vi "GyroDrive.vi"(0 "X axis value":dbl, 1 "Y axis value":dbl, 2 "RobotDriveDevRef_In":T1={"DevStatus"={"status"=FALSE, "code"=0, "source"=""}, "Motors[]"=[], "Square Inputs"=FALSE, "Max Output"=1.0}, 3 "Use gyro":bool, 4 "error in (no error)":errorcluster) -> (5 "Motor Values":dbl[](array[numeric]), 6 "RobotDriveDevRef_Out":T1={"DevStatus"={"status"=FALSE, "code"=0, "source"=""}, "Motors[]"=[], "Square Inputs"=FALSE, "Max Output"=1.0}, 7 "error out":errorcluster)   [LabVIEW 2015]
uses:
  <vilib>/Rock Robotics/WPI/RobotDrive/WPI_RobotDriveDevRef.ctl
  <vilib>/Rock Robotics/WPI/MotorControl/WPI_MotorControlDeviceRef.ctl
  <vilib>/Rock Robotics/WPI/MotorControl/WPI_MotorControlType.ctl
  <vilib>/Rock Robotics/SystemInterfaces/DIO/FPGA_DIOPWMChannel.ctl
  <vilib>/Rock Robotics/WPI/PWM/WPI_PWMDeadband.ctl
  <vilib>/Rock Robotics/WPI/CAN/Jaguar/SubVIs/WPI_CANJaguar_ControlMode.ctl
  <vilib>/Rock Robotics/WPI/CAN/TalonSRX/WPI_CANTalonSRX_APIControlMode.ctl
  Robot Global Data.vi
  <vilib>/Rock Robotics/WPI/RobotDrive/WPI_RobotDriveArcadeDrive_Standard(NoSaturation).vi
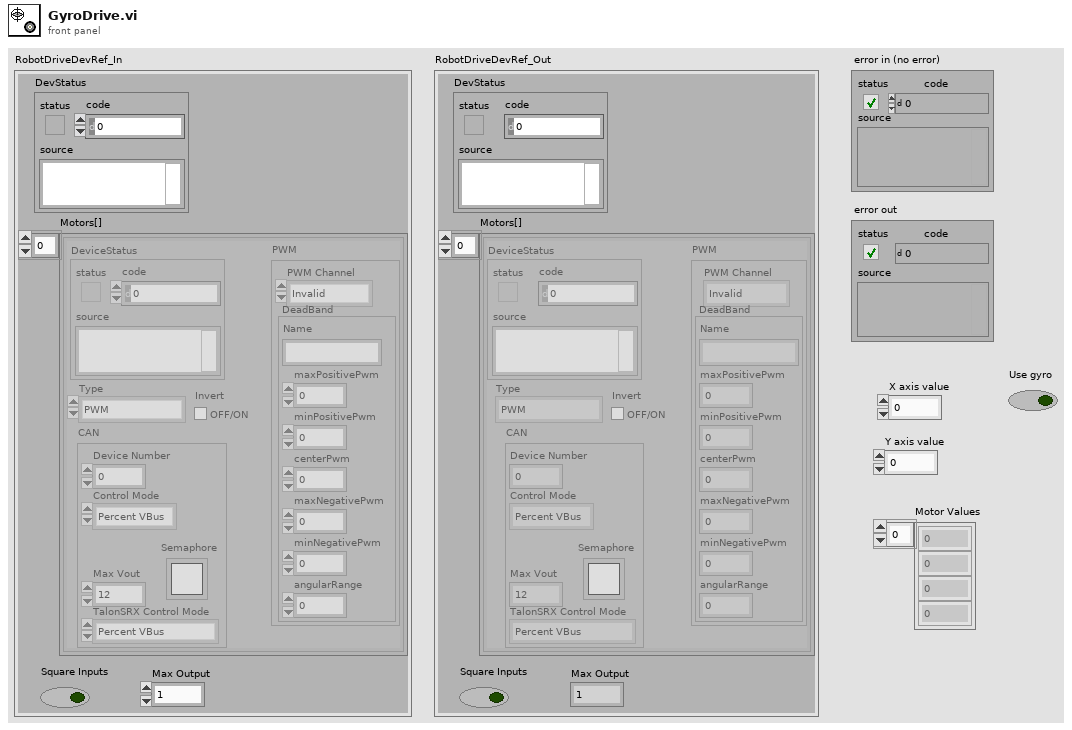
[diagram p1: front panel]
types:
  T1 = typedef "WPI_RobotDriveDevRef.ctl" = cluster{"DevStatus":errorcluster, "Motors[]":T2[], "Square Inputs":bool, "Max Output":dbl}
  T2 = typedef "WPI_MotorControlDeviceRef.ctl" = cluster{"DeviceStatus":errorcluster, "Type":T3, "PWM":cluster{"PWM Channel":T4, "DeadBand":T5}, "CAN":cluster{"Device Number":u8, "Control Mode":T6, "Semaphore":T7, "Max Vout":dbl, "TalonSRX Control Mode":T8}, "Invert":bool}
  T3 = typedef "WPI_MotorControlType.ctl" = enum16{"PWM", "CAN", "CANTalonSRX"}
  T4 = typedef "FPGA_DIOPWMChannel.ctl" = enum8{"PWM 0", "PWM 1", "PWM 2", "PWM 3", "PWM 4", "PWM 5", "PWM 6", "PWM 7", "PWM 8", "PWM 9", "PWM MXP 0", "PWM MXP 1", "PWM MXP 2", "PWM MXP 3", "PWM MXP 4", "PWM MXP 5", "PWM MXP 6", "PWM MXP 7", "PWM MXP 8", "PWM MXP 9", "Invalid"}
  T5 = typedef "WPI_PWMDeadband.ctl" = cluster{"Name":string, "maxPositivePwm":i32, "minPositivePwm":i32, "centerPwm":i32, "maxNegativePwm":i32, "minNegativePwm":i32, "angularRange":u16}
  T6 = typedef "WPI_CANJaguar_ControlMode.ctl" = enum8{"Percent VBus", "Current", "Speed", "Position", "Voltage"}
  T7 = typedef "Semaphore RefNum" = refnum<k1>
  T8 = typedef "WPI_CANTalonSRX_APIControlMode.ctl" = enum8{"Percent VBus", "Speed", "Position", "Slave", "Unchanged / Invalid", "Voltage Compensation", "Current", "Motion Profile"}
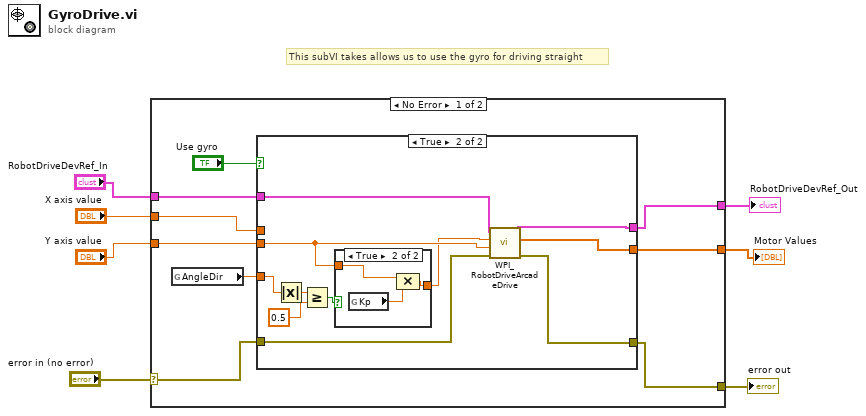
[diagram p0: block diagram]
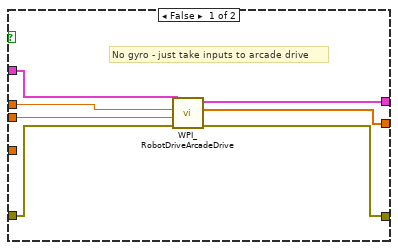
[diagram p2: hidden frame]
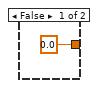
[diagram p3: hidden frame]
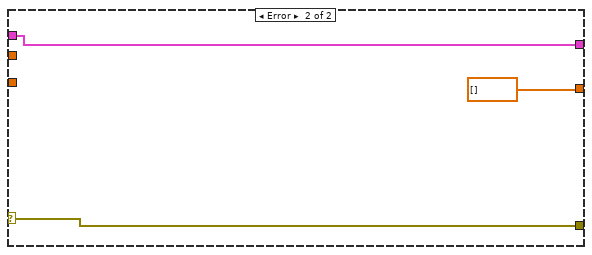
[diagram p4: hidden frame]
diagram:
  # "This subVI takes allows us to use the gyro for driving straight"
  n1 = case shown="No Error" "error in (no error)" {
    selector: "error in (no error)" -> [w13 w41]
    tunnel: [w12 w41] -> w6
    tunnel: "X axis value" -> [w16 _]
    tunnel: "Y axis value" -> [w15 _]
    tunnel: "RobotDriveDevRef_In" -> [w11 w40]
    tunnel: [w10 w40] -> w2
    tunnel: [w8 dbl[] [] ("Motor Values")] -> w1
    frame No Error {
      n2 = global read "Robot Global Data.vi" "AngleDir"() -> (w9:dbl)
      n3 = case shown="True" "Use gyro" {
        tunnel: w16 -> [w23 _]
        tunnel: w15 -> [w22 w29]
        tunnel: w13 -> [w21 w32]
        tunnel: [w20 w31] -> w12
        tunnel: w11 -> [w19 w33]
        tunnel: [w18 w34] -> w10
        tunnel: w9 -> [_ w24]
        tunnel: [w17 w30] -> w8
        frame False {
          # "No gyro - just take inputs to arcade drive"
          n4 = call-poly <vilib>:"WPI_RobotDriveArcadeDrive.vi"("error in (no error)"=w21, "Y axis value"=w22, "X axis value"=w23, "RobotDriveDevRef"=w19) -> ("error out"=w20:errorcluster, "Motor Values"=w17:dbl[], "RobotDriveDevRef"=w18:T1)  [unwired: 5 in]
        }
        frame True {
          n5 = Absolute Value(x=w24) -> (abs(x)=w26:dbl)
          n6 = Greater Or Equal?(x=w26, y=0.5) -> (x >= y?=w25:bool)
          n7 = case shown="True" w25 {
            tunnel: w29 -> [_ w38]
            tunnel: [0.0 w37] -> w28
            frame False {
            }
            frame True {
              n8 = global read "Robot Global Data.vi" "Kp"() -> (w36:dbl)
              n9 = Compound Arithmetic op=MULTIPLY(w38, w36) -> (w37:dbl)
            }
          }
          n10 = call-poly <vilib>:"WPI_RobotDriveArcadeDrive.vi"("error in (no error)"=w32, "Y axis value"=w29, "X axis value"=w28, "RobotDriveDevRef"=w33) -> ("error out"=w31:errorcluster, "Motor Values"=w30:dbl[], "RobotDriveDevRef"=w34:T1)  [unwired: 5 in]
        }
      }
    }
    frame Error {
    }
  }
  "error out" <- w6
  "RobotDriveDevRef_Out" <- w2
  "Motor Values" <- w1
